vi "RunCTRL.vi"(8 "error in (no error)":errorcluster) -> (0 "error out":errorcluster)   [LabVIEW 2017, in "programControl.lvlib"]
doc: "This is the main Program Control VI. It is responsible for starting and stopping all the other module main VIs."
uses:
  programControl.lvlib
  TypeDefs/programControlStates.ctl
  UEFGV/Type Def/UEFGV_States.ctl
  loggingModule/Queue/TypeDefs/message.ctl
  <vilib>/event_ctls.llb/usereventprio.ctl
  ErrorMonitor/ErrorMonitor.lvlib
  loggingModule/loggingModule.lvlib
panel:
  out "Shutdown":bool
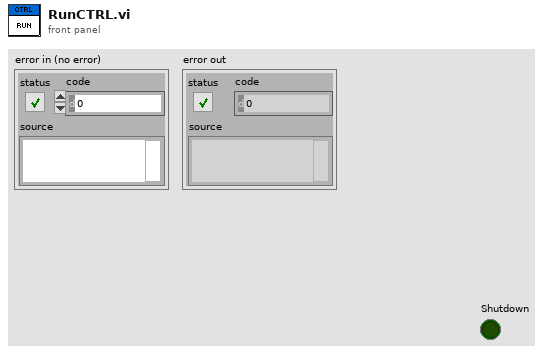
[diagram p1: front panel]
types:
  T1 = typedef "UEFGV_States.ctl" = enum16{"Create", "Get", "Destroy"}
  T2 = typedef "programControl.lvlib/programControlStates.ctl" = enum16{"init", "run", "shutdown"}
  T3 = typedef "loggingModule.lvlib/message.ctl" = cluster{"calling module":string, "message":string, "data":variant}
  T4 = typedef "usereventprio.ctl" = enum32{"high priority", "normal priority"}
  T5 = typedef "programControl.lvlib/message.ctl" = cluster{"calling module":string, "message":string, "Data":variant}
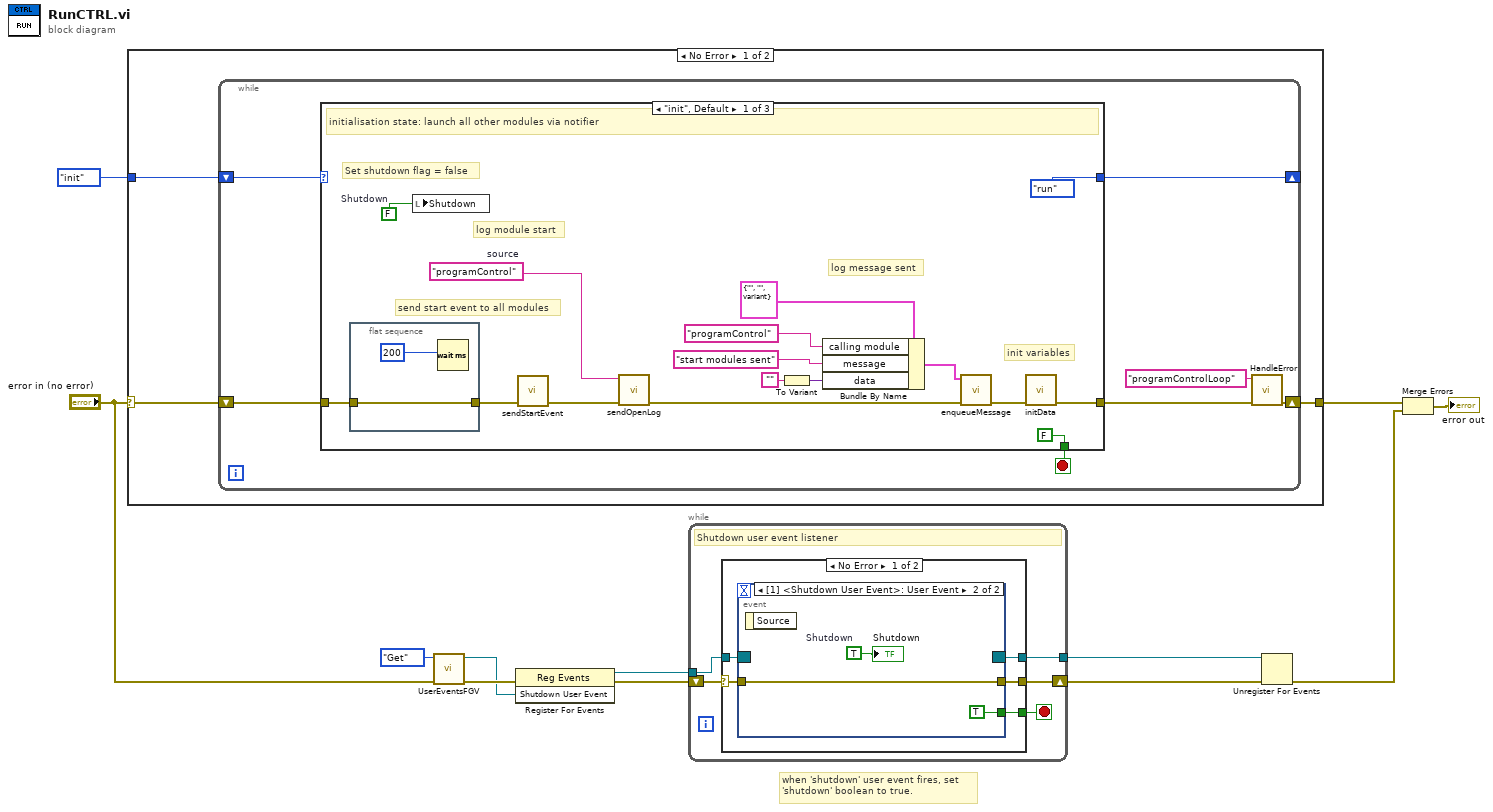
[diagram p0: block diagram]
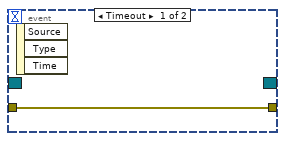
[diagram p2: hidden frame]
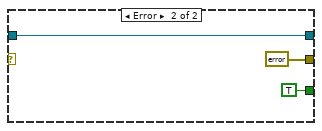
[diagram p3: hidden frame]
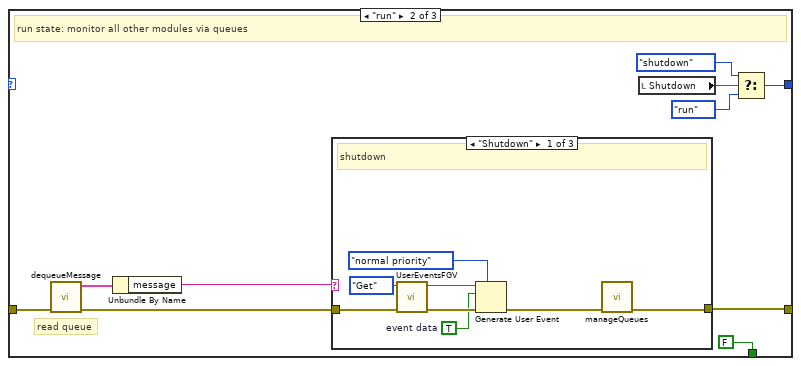
[diagram p4: hidden frame]
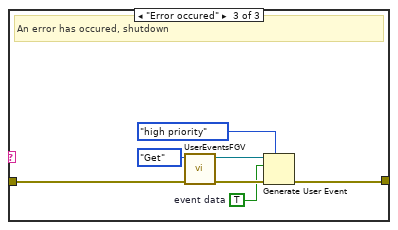
[diagram p6: hidden frame]
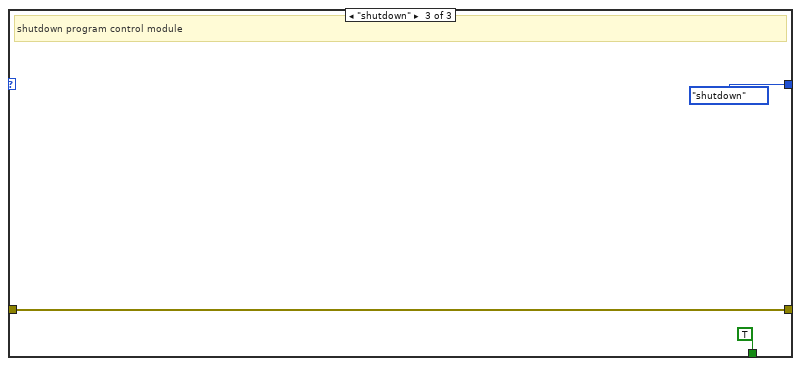
[diagram p7: hidden frame]
diagram:
  # "when 'shutdown' user event fires, set\n'shutdown' boolean to true."
  n1 = case shown="No Error" "error in (no error)" {
    selector: "error in (no error)" -> [w15 w70]
    tunnel: [w14 w70] -> w4
    tunnel: programControlStates."init" -> [w13 _]
    frame No Error {
      n2 = while {
        shift-right: [w21] -> _
        shift-left: w13 -> [w22]
        shift-right: [w17] -> w14
        shift-left: w15 -> [w19]
        stop <- w20 stop-if-true
        n3 = case shown="\"init\", Default" w22 {
          tunnel: [programControlStates."run" w47 programControlStates."shutdown"] -> w21
          tunnel: [FALSE FALSE TRUE] -> w20
          tunnel: [w27 w44 w67] -> w18
          tunnel: w19 -> [w25 w46 w67]
          frame "init", Default {
            w29 = "programControl"  # source
            w36 = FALSE  # Shutdown
            # "init variables"
            # "log module start"
            # "send start event to all modules"
            # "Set shutdown flag = false"
            # "log message sent"
            # "initialisation state: launch all other modules via notifier"
            n4 = flat-sequence {
              tunnel: w25 -> [w39]
              tunnel: [w39] -> w24
              frame #0 {
                n5 = Wait (ms)(milliseconds to wait=u32 200) -> ()  [unwired: 1 out]
              }
            }
            n6 = local write "Shutdown"(w36) -> ()
            n7 = call "sendStartEvent.vi"("error in (no error)"=w24) -> ("error out"=w26:errorcluster)  [unwired: 10 in]
            n8 = call "sendOpenLog.vi"("error in (no error)"=w26, "source"=w29) -> ("error out"=w30:errorcluster)  [unwired: 9 in]
            n9 = To Variant(anything="") -> (Variant=w31:variant)
            n10 = Bundle By Name(cluster=T3 {"calling module"="", "message"="", "data"=variant} ("message in"), "calling module"="programControl", "message"="start modules sent", "data"=w31) -> (w23:T3)
            n11 = call "enqueueMessage.vi"("error in (no error)"=w30, "Message"=w23) -> ("error out"=w28:errorcluster)  [unwired: 9 in]
            n12 = call "initData.vi"("error in (no error)"=w28) -> ("error out"=w27:errorcluster)  [unwired: 10 in]
          }
          frame "run" {
            # "read queue"
            # "run state: monitor all other modules via queues"
            n13 = call "dequeueMessage.vi"("error in (no error)"=w46) -> ("error out"=w45:errorcluster, "element"=w42:T5)  [unwired: 9 in]
            n14 = Unbundle By Name(w42) -> ("message"=w41:string)
            n15 = case shown="\"Shutdown\"" w41 {
              tunnel: w45 -> [w53 w59 w62]
              tunnel: [w51 w59 w61] -> w44
              frame "Shutdown" {
                w54 = TRUE  # event data
                # "shutdown"
                n16 = call "UserEventsFGV.vi"("error in (no error)"=w53, "Command"=UEFGV_States."Get") -> ("error out"=w58:errorcluster, "Shutdown User Event"=w57:refnum<user-event>)  [unwired: 8 in]
                n17 = Generate User Event(priority (normal)=usereventprio."normal priority", user event=w57, event data cluster=w54, error in=w58) -> (error out=w52:errorcluster)  [unwired: 1 out]
                n18 = call "manageQueues.vi"("error in (no error)"=w52) -> ("error out"=w51:errorcluster)  [unwired: 10 in]
              }
              frame "wait", Default {
                # "Do nothing"
              }
              frame "Error occured" {
                w60 = TRUE  # event data
                # "An error has occured, shutdown"
                n19 = call "UserEventsFGV.vi"("error in (no error)"=w62, "Command"=UEFGV_States."Get") -> ("error out"=w66:errorcluster, "Shutdown User Event"=w65:refnum<user-event>)  [unwired: 8 in]
                n20 = Generate User Event(priority (normal)=usereventprio."high priority", user event=w65, event data cluster=w60, error in=w66) -> (error out=w61:errorcluster)  [unwired: 1 out]
              }
            }
            n21 = local read "Shutdown"() -> (w43:bool)
            n22 = Select(t=programControlStates."shutdown", s=w43, f=programControlStates."run") -> (s? t:f=w47:T2)
          }
          frame "shutdown" {
            # "shutdown program control module"
          }
        }
        n23 = call "HandleError.vi"("error in (no error)"=w18, "Source"="programControlLoop") -> ("error out"=w17:errorcluster)  [unwired: 9 in]
      }
    }
    frame Error {
    }
  }
  n24 = call "UserEventsFGV.vi"("error in (no error)"="error in (no error)", "Command"=UEFGV_States."Get") -> ("error out"=w9:errorcluster, "Shutdown User Event"=w8:refnum<user-event>)  [unwired: 8 in]
  n25 = register-events(error in=w9, w8) -> (reference out=w11:refnum<event-registration>, error out=w6:errorcluster)  [unwired: 1 in]
  n26 = while {
    tunnel: w11 -> [w75]
    tunnel: [w74] -> w10
    shift-right: [w71] -> w7
    shift-left: w6 -> [w72]
    stop <- w73 stop-if-true
    # "Shutdown user event listener"
    n27 = case shown="No Error" w72 {
      selector: w72 -> [w77 _]
      tunnel: w75 -> [w80 w86]
      tunnel: [w79 w86] -> w74
      tunnel: [w78 TRUE] -> w73
      tunnel: [w76 errorcluster {"status"=FALSE, "code"=0, "source"=""} ("error out")] -> w71
      frame No Error {
        n28 = event shown="[1] <Shutdown User Event>: User Event" {
          selector: w80 -> [_ _]
          dyn-events: [_ _] -> w79
          timeout: _ -> [_ _]
          tunnel: w77 -> [w81 w83]
          tunnel: [w81 w83] -> w76
          tunnel: [_ TRUE] -> w78
          event Timeout {
            n29 = event-data() -> ()  [unwired: 1 in, 3 out]
          }
          event User Event {
            w82 = TRUE  # Shutdown
            n30 = event-data() -> ()  [unwired: 1 in, 1 out]
            "Shutdown" <- w82
          }
        }
      }
      frame Error {
      }
    }
  }
  n31 = Unregister For Events(event registration refnum=w10, error in=w7) -> (error out=w3:errorcluster)
  n32 = Merge Errors(w4, w3) -> (→"error out":errorcluster)
